vi "nonlinear filter.vi"(0 "p12":dbl, 5 "p21":dbl, 7 "soft":dbl) -> (4 "p12":dbl, 8 "bit":bool)   [LabVIEW 2017]
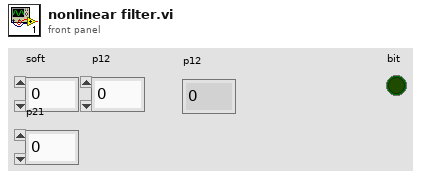
[diagram p1: front panel]
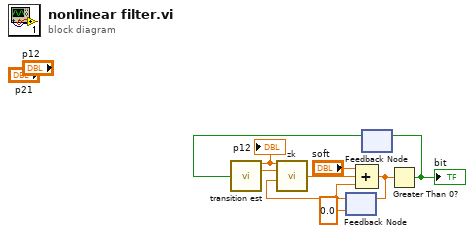
[diagram p0: block diagram]
diagram:
  n1 = feedback #1(0.0) -> (w6:dbl)
  n2 = feedback #2() -> (w3:bool)  [unwired: 1 in]
  n3 = call "transition est.vi"("bit"=w3) -> ("p12"=w2:dbl, "p21"=w1:dbl)  [unwired: 13 in]
  "p12" <- w2
  n4 = call "zk.vi"("p12"=w2, "p21"=w1, "uk"=w6) -> ("zk"=w7:dbl)  [unwired: 12 in]
  n5 = Compound Arithmetic op=ADD("soft", w7, w6) -> (w8:dbl)
  n6 = feedback-in #1(w8) -> ()
  n7 = Greater Than 0?(x=w8) -> (x > 0?=w4:bool)
  "bit" <- w4
  n8 = feedback-in #2(w4) -> ()
